vi "Mask with NaN.vi"(2 "Mask":dbl[](array[numeric]), 3 "Array IN":dbl[](array[numeric])) -> (0 "Array OUT":dbl[](array[numeric]))   [LabVIEW 2013, in "nan operations.lvlib"]
uses:
  nan operations.lvlib
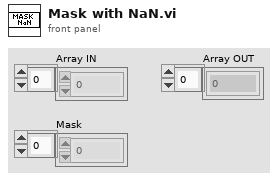
[diagram p1: front panel]
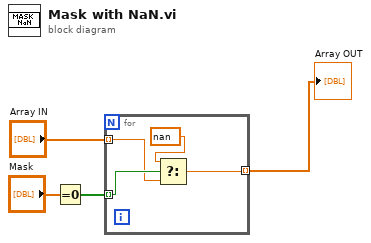
[diagram p0: block diagram]
diagram:
  n1 = Equal To 0?(x="Mask") -> (x = 0?=w3:bool[])
  n2 = for {
    tunnel: w3 -> [w8] mode=indexing
    tunnel: "Array IN" -> [w7] mode=indexing
    tunnel: [w5] -> w1 mode=indexing
    n3 = Select(t=nan, s=w8, f=w7) -> (s? t:f=w5:dbl)
  }
  "Array OUT" <- w1
